vi "Interpolation Test.vi"() -> ()   [LabVIEW 2014]
uses:
  <vilib>/rvi/interface/nirviMethod/nirviMethod.xnode
  <vilib>/FPGAPlugInAG/Dynamic/niLvFpga_Abort_Dynamic.vi
  <vilib>/rvi/interface/nirviCloseFPGA/nirviCloseFPGA.xnode
  <vilib>/FPGAPlugInAG/Dynamic/niLvFpga_Close_Dynamic.vi
panel:
  out "Max Amp":fxp<+,46,22>
  out "Max Bin":i32
  in  "stop":bool
  out "Detected Frequency (Hz)":dbl
  in  "Sample Rate (S/s)":dbl=50000000.0 format="%#_13g"
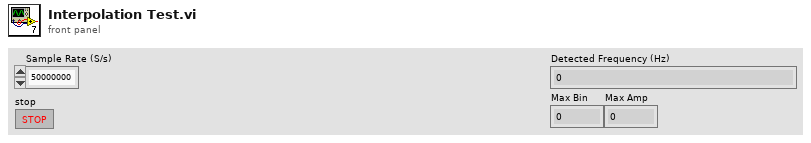
[diagram p1: front panel]
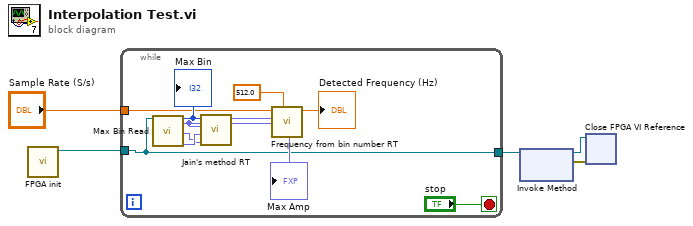
[diagram p0: block diagram]
diagram:
  n1 = call "FPGA init.vi"() -> ("FPGA VI Reference Out"=w2:refnum<k20>)  [unwired: 10 in, 1 out]
  n2 = while {
    tunnel: w2 -> [w6]
    tunnel: "Sample Rate (S/s)" -> [w10]
    tunnel: [w6] -> w1
    stop <- "stop" stop-if-true
    n3 = call "Max Bin Read.vi"("FPGA VI Reference In"=w6) -> ("Max Bin"=w15:i32, "Max Amp"=w14:fxp<+,46,22>, "Prev Amp"=w7:fxp<+,46,22>, "Next Amp"=w8:fxp<+,46,22>)  [unwired: 13 in, 2 out]
    "Max Bin" <- w15
    "Max Amp" <- w14
    n4 = call "Jain's method RT.vi"("Prev Amp"=w7, "Next Amp"=w8, "Max Amp"=w14, "Max Bin"=w15) -> ("Bin"=w9:fxp<+/-,64,66>)  [unwired: 7 in]
    n5 = call "Frequency from bin number RT.vi"("FFT size"=512.0, "Bin number"=w9, "Sample Rate (S/s)"=w10) -> ("Detected Frequency (Hz)"=→"Detected Frequency (Hz)":dbl)  [unwired: 8 in]
  }
  n6 = xnode "Invoke Method"("FPGA VI Reference In"=w1) -> ("FPGA VI Reference Out"=w4:refnum<k20>, "error out"=w3:errorcluster)  [unwired: 1 in]
  n7 = xnode "Close FPGA VI Reference"("FPGA VI Reference In"=w4, "error in"=w3) -> ()  [unwired: 1 out]
